vi "Chebyshev Approximation Prep.vi"(4 "start":dbl format="%.2f", 7 "formula":string, 8 "end":dbl format="%.2f") -> (0 "value 2":dbl format="%.2f", 1 "Parsed Formula":cluster{"Table":i32[][], "Y Values":dbl[]} {"Y Values" format="%.2f"}, 2 "value 1":dbl format="%.2f", 3 "error (general)":bool, 5 "x string":string, 6 "error situation":bool)   [LabVIEW 2018, in "NI_Gmath.lvlib"]
uses:
  NI_Gmath.lvlib
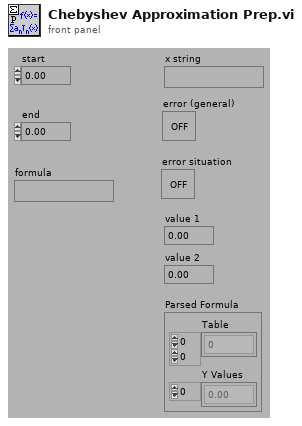
[diagram p1: front panel]
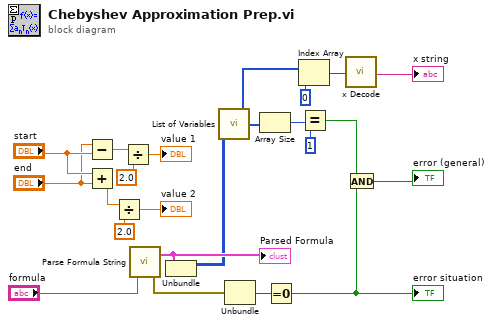
[diagram p0: block diagram]
diagram:
  n1 = Subtract(x="end", y="start") -> (x-y=w1:dbl)
  n2 = Add(x="start", y="end") -> (x+y=w6:dbl)
  n3 = Divide(x=w6, y=2.0) -> (x/y=→"value 2":dbl)
  n4 = Divide(x=w1, y=2.0) -> (x/y=→"value 1":dbl)
  n5 = call "Parse Formula String.vi"("formula"="formula") -> ("error out"=w16:errorcluster, "Parsed Formula"=w22:cluster{"Table":i32[][], "Y Values":dbl[]})  [unwired: 1 in]
  "Parsed Formula" <- w22
  n6 = Unbundle(w22) -> ("Table"=w21:i32[][])  [unwired: 1 out]
  n7 = call "List of Variables.vi"("Table"=w21) -> ("List of variables"=w10:i32[])
  n8 = Unbundle(w16) -> ("code"=w17:i32)  [unwired: 2 out]
  n9 = Array Size(array=w10) -> (size(s)=w11:i32)
  n10 = Equal To 0?(x=w17) -> (x = 0?=w20:bool)
  "error situation" <- w20
  n11 = Index Array(array=w10, index=0) -> (element=w15:i32)
  n12 = Equal?(x=w11, y=1) -> (x = y?=w18:bool)
  n13 = call "x Decode.vi"("number"=w15) -> ("x string"=→"x string":string)  [unwired: 1 in, 1 out]
  n14 = And(x=w18, y=w20) -> (x .and. y?=→"error (general)":bool)
